vi "model-TRABS.vi"(2 "BG":dbl=-0.0001 format="%#_13g", 3 "Real delay time, ps":dbl) -> (0 "signal out":dbl[](array[numeric]))   [LabVIEW 2015]
uses:
  globalVarSD.vi
panel:
  in  "x":dbl
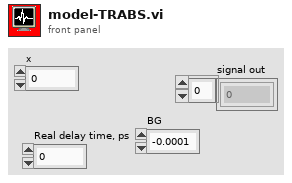
[diagram p1: front panel]
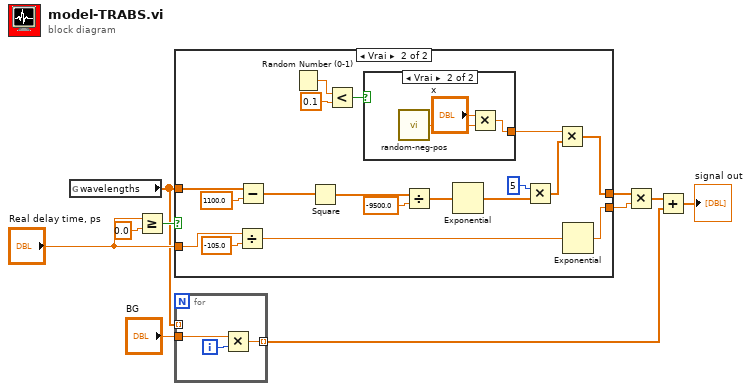
[diagram p0: block diagram]
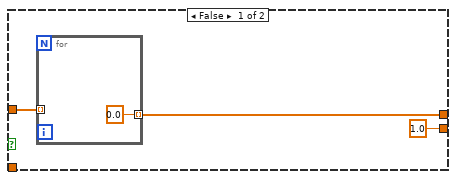
[diagram p2: hidden frame]
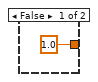
[diagram p3: hidden frame]
diagram:
  n1 = global read "globalVarSD.vi" "wavelengths"() -> (w1:dbl[])
  n2 = Greater Or Equal?(x="Real delay time, ps", y=0.0) -> (x >= y?=w9:bool)
  n3 = case shown="Vrai" w9 {
    tunnel: [1.0 w30] -> w8
    tunnel: "Real delay time, ps" -> [_ w29]
    tunnel: w1 -> [w12 w23]
    tunnel: [w11 w15] -> w6
    frame False {
      n4 = for {
        tunnel: w12 -> [_] mode=indexing
        tunnel: [0.0] -> w11 mode=indexing
      }
    }
    frame True {
      n5 = Divide(x=w29, y=-105.0 ("tau")) -> (x/y=w31:dbl)
      n6 = Subtract(x=w23, y=1100.0 ("x0")) -> (x-y=w27:dbl[])
      n7 = Random Number (0-1)() -> (number: 0 to 1=w20:dbl)
      n8 = Square(x=w27) -> (x^2=w26:dbl[])
      n9 = Less?(x=w20, y=0.1) -> (x < y?=w18:bool)
      n10 = case shown="Vrai" w18 {
        tunnel: [1.0 w36] -> w16
        frame False {
        }
        frame True {
          n11 = call "random-neg-pos.vi"() -> ("out"=w35:dbl)
          n12 = Multiply(x="x", y=w35) -> (x*y=w36:dbl)
        }
      }
      n13 = Divide(x=w26, y=-9500.0 ("sig,q")) -> (x/y=w25:dbl[])
      n14 = Exponential(1:w25) -> (0:w22:dbl[])
      n15 = Multiply(x=5, y=w22) -> (x*y=w17:dbl[])
      n16 = Multiply(x=w16, y=w17) -> (x*y=w15:dbl[])
      n17 = Exponential(1:w31) -> (0:w30:dbl)
    }
  }
  n18 = for {
    tunnel: "BG" -> [w38]
    tunnel: [w37] -> w2 mode=indexing
    tunnel: w1 -> [_] mode=indexing
    i -> [w39]
    n19 = Multiply(x=w38, y=w39) -> (x*y=w37:dbl)
  }
  n20 = Multiply(x=w6, y=w8) -> (x*y=w5:dbl[])
  n21 = Add(x=w5, y=w2) -> (x+y=→"signal out":dbl[])
